vi "I32_I8.vi"(4 "x":i32) -> (1 "数组":i8[](array[numeric]) format="%x")   [LabVIEW 2019]
panel:
  out "i":u8
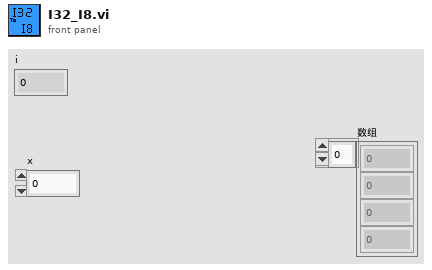
[diagram p1: front panel]
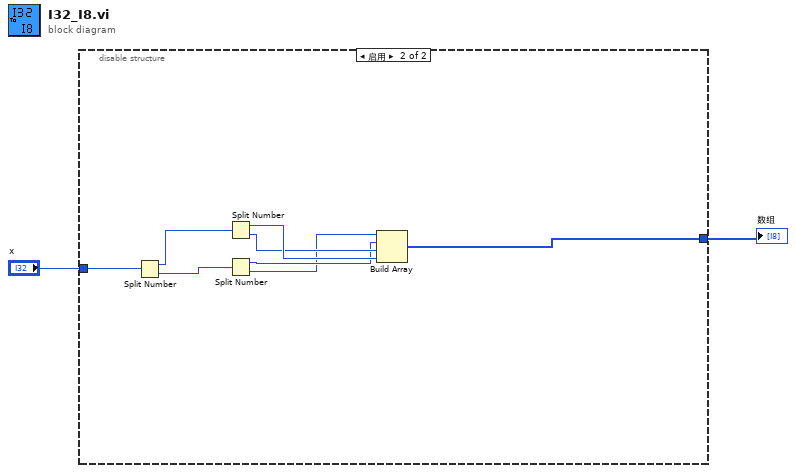
[diagram p0: block diagram]
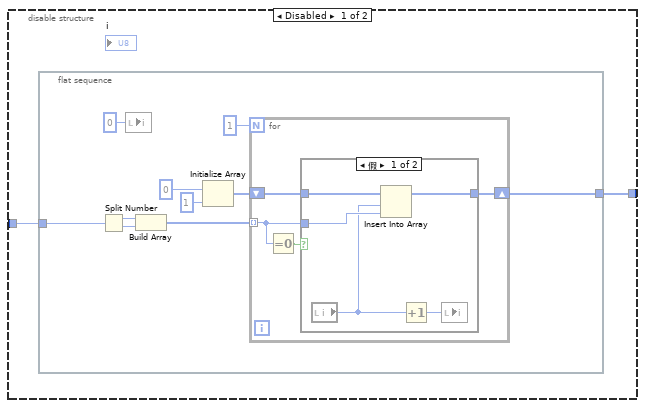
[diagram p2: hidden frame]
diagram:
  n1 = disable-structure shown="启用" {
    disable-tunnel: "x" -> [w4 w32]
    disable-tunnel: [w3 w31] -> w1
    frame Disabled {
      n2 = flat-sequence {
        tunnel: w4 -> [w6]
        tunnel: [w5] -> w3
        frame #0 {
          n3 = Split Number(x=w6) -> (hi(x)=w8:u16, lo(x)=w7:u16)
          n4 = local write "i"(u8 0 ("i")) -> ()
          n5 = Build Array(w8, w7) -> (w13:u16[])
          n6 = Initialize Array(i8 0 ("元素"), 1 ("维数大小")) -> (w10:i8[])
          n7 = for {
            N: 1 -> [_]
            tunnel: w13 -> [w17] mode=indexing
            shift-right: [w16] -> w5
            shift-left: w10 -> [w15]
            n8 = Equal To 0?(x=w17) -> (x = 0?=w18:bool)
            n9 = case shown="假" w18 {
              tunnel: w17 -> [w22 _]
              tunnel: [w20 w24] -> w16
              tunnel: w15 -> [w19 w24]
              frame False {
                n10 = local read "i"() -> (w21:u8)
                n11 = Insert Into Array(array=w19, index=w21, new element=w22) -> (w20:i8[])
                n12 = Increment(x=w21) -> (x+1=w23:u8)
                n13 = local write "i"(w23) -> ()
              }
              frame True {
              }
            }
          }
        }
      }
    }
    frame Enabled {
      n14 = Split Number(x=w32) -> (hi(x)=w30:u16, lo(x)=w29:u16)
      n15 = Split Number(x=w30) -> (hi(x)=w28:u8, lo(x)=w27:u8)
      n16 = Split Number(x=w29) -> (hi(x)=w26:u8, lo(x)=w25:u8)
      n17 = Build Array(w25, w26, w27, w28) -> (w31:u8[])
    }
  }
  "数组" <- w1
